vi "MPG Sandbox.vi"() -> ()   [LabVIEW 2011]
uses:
  Gantry Class.lvclass
panel:
  in  "Config Folder":path=path "C:/Users/Husker/Desktop/gantry/Config"
  out "error out":errorcluster
  in  "stop":bool
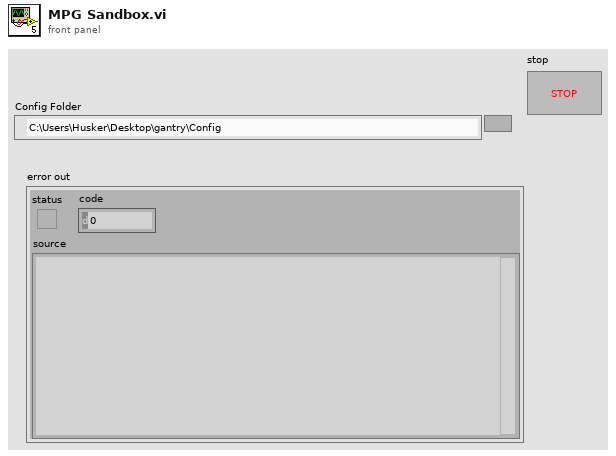
[diagram p1: front panel]
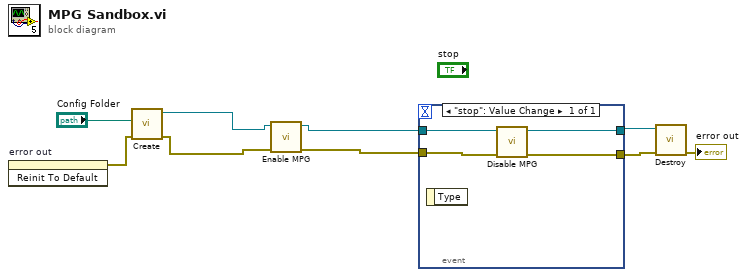
[diagram p0: block diagram]
diagram:
  n1 = invoke on="error out" class="Clust (strict)" method="Reinit To Default"() -> (error out=w7:errorcluster)  [unwired: 3 in, 2 out]
  n2 = call "Create.vi"("error in (no error)"=w7, "Config Folder"="Config Folder") -> ("error out"=w3:errorcluster, "Gantry Class out"=w4:refnum<class "Gantry Class.lvclass">)  [unwired: 8 in]
  n3 = call-dynamic "Enable MPG.vi"("error in (no error)"=w3, "Gantry Class in"=w4) -> ("error out"=w1:errorcluster, "Gantry Class out"=w2:refnum<class "Gantry Class.lvclass">)  [unwired: 8 in]
  n4 = event shown="[0] \"stop\": Value Change" {
    selector: _ -> [_]
    dyn-events: _ -> [_]
    timeout: _ -> [_]
    tunnel: w2 -> [w12]
    tunnel: [w13] -> w6
    tunnel: [w10] -> w5
    tunnel: w1 -> [w11]
    event "stop": Value Change {
      n5 = event-data() -> ()  [unwired: 1 in, 1 out]
      n6 = call-dynamic "Disable MPG.vi"("error in (no error)"=w11, "Gantry Class in"=w12) -> ("error out"=w10:errorcluster, "Gantry Class out"=w13:refnum<class "Gantry Class.lvclass">)  [unwired: 8 in]
    }
  }
  n7 = call "Destroy.vi"("error in (no error)"=w5, "Gantry Class in"=w6) -> ("error out"=→"error out":errorcluster)  [unwired: 9 in]
